vi "open_dyn_PrepLineObjects_window.vi"(8 "error in (no error)":errorcluster) -> (0 "error out":errorcluster)   [LabVIEW 2018]
doc: "dynamically opens the window that shows the PrepLineObjects"
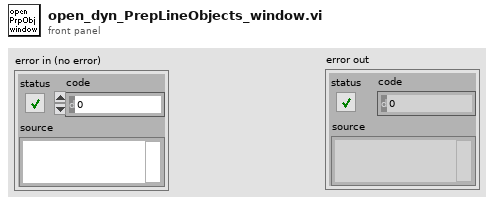
[diagram p1: front panel]
types:
  T1 = enum32{"Invalid", "Standard", "Closed", "Hidden", "Minimized", "Maximized"}
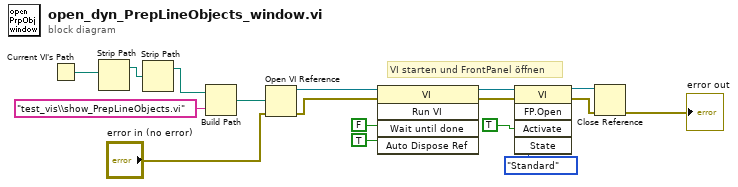
[diagram p0: block diagram]
diagram:
  # "VI starten und FrontPanel öffnen"
  n1 = Current VI's Path() -> (path=w3:path)
  n2 = Strip Path(path=w3) -> (stripped path=w2:path)  [unwired: 1 out]
  n3 = Strip Path(path=w2) -> (stripped path=w1:path)  [unwired: 1 out]
  n4 = Build Path(base path=w1, name or relative path="test_vis\\show_PrepLineObjects.vi") -> (appended path=w9:path)
  n5 = Open VI Reference(vi path=w9, error in (no error)="error in (no error)") -> (vi reference=w5:refnum<vi>, error out=w4:errorcluster)  [unwired: 4 in]
  n6 = invoke class="VI" method="Run VI"(reference=w5, error in=w4, "Wait until done"=FALSE, "Auto Dispose Ref"=TRUE) -> (reference out=w15:refnum<vi>, error out=w14:errorcluster)  [unwired: 1 in, 3 out]
  n7 = invoke class="VI" method="FP.Open"(reference=w15, error in=w14, "Activate"=TRUE, "State"=T1."Standard") -> (reference out=w11:refnum<vi>, error out=w10:errorcluster)  [unwired: 1 in, 3 out]
  n8 = Close Reference(reference=w11, error in (no error)=w10) -> (error out=→"error out":errorcluster)
